vi "Send Log Data.vi"(8 "error in":errorcluster, 10 "Data":T1[](array[typedef]) {"type" format="%04x"; "activity" format="%04x"; "error" format="%04x"; "cwd1" format="%04x"; "cwd2" format="%04x"; "swd1" format="%04x"; "swd2" format="%04x"; "data" format="%04x"}, 11 "Producer in":refnum<class "Log Producer.lvclass">) -> (0 "error out":errorcluster, 3 "Producer out":refnum<class "Log Producer.lvclass">)   [LabVIEW 2020, in "AIM MIL-STD-1553 Engine.lvlib" / "Implementation.lvlib" / "Word Logging.lvlib"]
uses:
  Word Logging.lvlib
  Log Producer/Log Producer.lvclass
  Word.ctl
  Implementation.lvlib
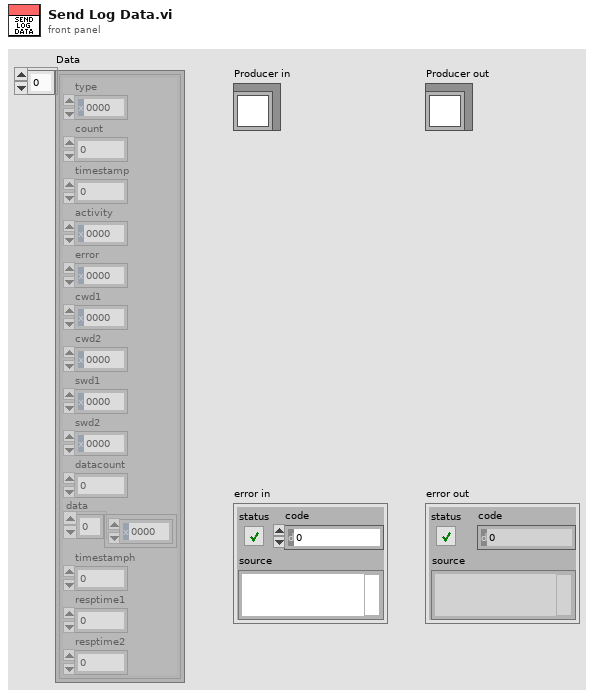
[diagram p1: front panel]
types:
  T1 = typedef "AIM MIL-STD-1553 Engine.lvlib/Implementation.lvlib/Word.ctl" = cluster{"type":u16, "count":u16, "timestamp":u32, "activity":u16, "error":u16, "cwd1":u16, "cwd2":u16, "swd1":u16, "swd2":u16, "datacount":u16, "data":u16[], "timestamph":u32, "resptime1":u16, "resptime2":u16}
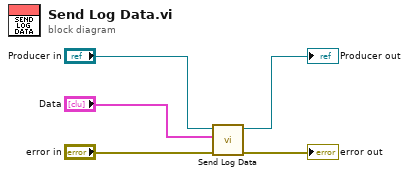
[diagram p0: block diagram]
diagram:
  n1 = call "Send Log Data.vi"("error in"="error in", "Data"="Data", "Log Producer in"="Producer in") -> ("error out"=→"error out":errorcluster, "Log Producer out"=→"Producer out":refnum<class "Log Producer.lvclass">)  [unwired: 7 in]
